vi "WriteRead.vi"(8 "error in (no error)":errorcluster, 10 "Command":string, 11 "Serial in":refnum<class "Serial.lvclass">) -> (0 "error out":errorcluster, 2 "Response":string, 3 "Serial out":refnum<class "Serial.lvclass">)   [LabVIEW 2014, in "Serial.lvclass"]
uses:
  Serial.lvclass
  Serial.lvclass/Serial.ctl
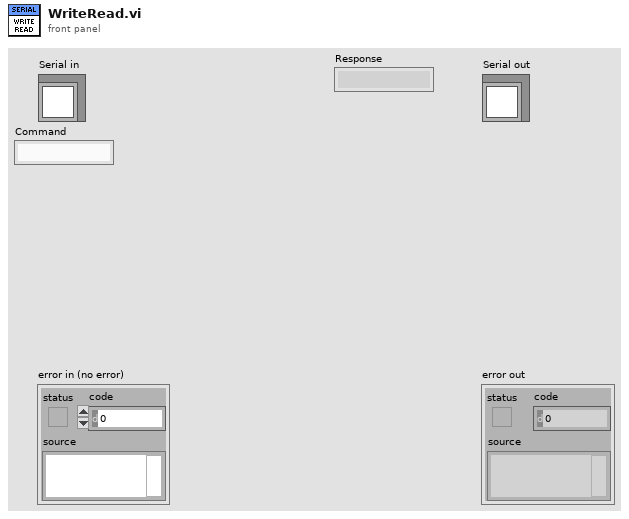
[diagram p1: front panel]
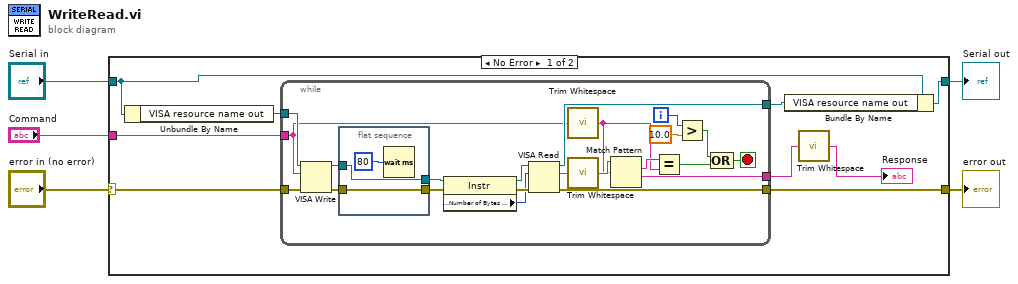
[diagram p0: block diagram]
diagram:
  n1 = case shown="No Error" "error in (no error)" {
    selector: "error in (no error)" -> [w13 w41]
    tunnel: [w12 w41] -> w4
    tunnel: [w10 w40] -> w2
    tunnel: "Serial in" -> [w11 w40]
    tunnel: "Command" -> [w8 _]
    frame No Error {
      n2 = Unbundle By Name(w11) -> ("VISA resource name out"=w14:refnum<visa-resource-name>)
      n3 = while {
        tunnel: w14 -> [w36]
        tunnel: w13 -> [w35]
        tunnel: [w34] -> w9
        tunnel: [w33] -> w12
        tunnel: w8 -> [w21]
        tunnel: [w29] -> w7
        i -> [w19]
        stop <- w16 stop-if-true
        n4 = VISA Write(VISA resource name=w36, write buffer=w21, error in (no error)=w35) -> (VISA resource name out=w27:refnum<visa-resource-name>, error out=w24:errorcluster)  [unwired: 1 out]
        n5 = flat-sequence {
          tunnel: [w39] -> w26
          tunnel: w27 -> [w39]
          tunnel: w24 -> [w38]
          tunnel: [w38] -> w25
          frame #0 {
            n6 = Wait (ms)(milliseconds to wait=u32 80) -> ()  [unwired: 1 out]
          }
        }
        n7 = property class="Instr"(reference=w26, error in=w25) -> (reference out=w32:refnum<visa-resource-name>, error out=w31:errorcluster, "Serial Settings:Number of Bytes at Serial Port"=w30:u32)
        n8 = VISA Read(VISA resource name=w32, byte count=w30, error in (no error)=w31) -> (VISA resource name out=w34:refnum<visa-resource-name>, read buffer=w23:string, error out=w33:errorcluster)  [unwired: 1 out]
        n9 = call <vilib>:"Trim Whitespace.vi"("string"=w21) -> ("trimmed string"=w15:string)  [unwired: 1 in]
        n10 = call <vilib>:"Trim Whitespace.vi"("string"=w23) -> ("trimmed string"=w22:string)  [unwired: 1 in]
        n11 = Match Pattern(string=w22, regular expression=w15) -> (match substring=w28:string, after substring=w29:string)  [unwired: 1 in, 2 out]
        n12 = Equal?(x=w28, y=w15) -> (x = y?=w17:bool)
        n13 = Greater?(x=w19, y=10.0) -> (0:w18:bool)
        n14 = Compound Arithmetic op=OR(w18, w17) -> (w16:bool)
      }
      n15 = Bundle By Name(cluster=w11, "VISA resource name out"=w9) -> (w10:refnum<class "Serial.lvclass">)
      n16 = call <vilib>:"Trim Whitespace.vi"("string"=w7) -> ("trimmed string"=→"Response":string)  [unwired: 1 in]
    }
    frame Error {
    }
  }
  "error out" <- w4
  "Serial out" <- w2
